vi "qFED.vi"(0 "System no.":i32=1 min=1 max=4 step=1, 2 "Axes to query":string[](array[string]), 3 "All axes?":bool, 4 "Axis identifier?":bool, 5 "error in":errorcluster) -> (14 "Edge ID":i32[](array[numeric]), 15 "Parameter":dbl[](array[numeric]), 19 "error out":errorcluster)   [LabVIEW 2026]
doc: "Get the parameters of the last Find Edge motion performed with FED.\n\nC-843: If All axes? = TRUE, then Axis identifier? can be FALSE"
panel:
  # "Get the parameters of the last Find Edge motion performed with FED."
  # "If all axes: use"
  # "Query"
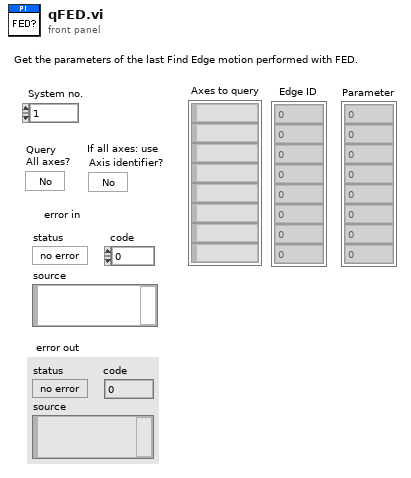
[diagram p1: front panel]
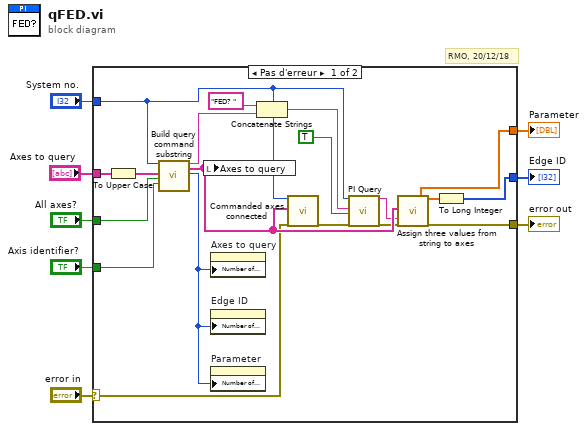
[diagram p0: block diagram]
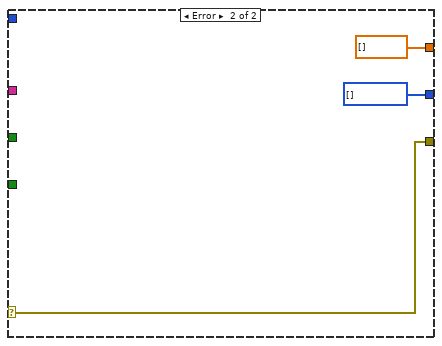
[diagram p2: hidden frame]
diagram:
  # "RMO, 20/12/18"
  n1 = case shown="Pas d'erreur" "error in" {
    selector: "error in" -> [w12 w28]
    tunnel: "Axes to query" -> [w25 _]
    tunnel: "System no." -> [w11 _]
    tunnel: [w27 w28] -> w6
    tunnel: [w15 i32[] [] ("Parameter values")] -> w5
    tunnel: [w14 dbl[] [] ("Source ID")] -> w4
    tunnel: "All axes?" -> [w24 _]
    tunnel: "Axis identifier?" -> [w23 _]
    frame No Error {
      n2 = To Upper Case(1:w25) -> (0:w26:string[])
      n3 = call "Build query command substring.vi"("System no."=w11, "Axes to query in"=w26, "Query\nAll axes?"=w24, "For all axes: use\nAxis identifier?"=w23) -> ("Command substring"=w18:string, "Axes to query out"=w13:string[], "Number of rows"=w22:u32)  [unwired: 2 in, 11 out]
      n4 = local write "Axes to query"(w13) -> ()
      n5 = property on="Axes to query" class="Tabl (strict)"("Number of Rows"=w22) -> ()  [unwired: 2 in, 2 out]
      n6 = property on="Edge ID" class="Tabl (strict)"("Number of Rows"=w22) -> ()  [unwired: 2 in, 2 out]
      n7 = property on="Parameter" class="Tabl (strict)"("Number of Rows"=w22) -> ()  [unwired: 2 in, 2 out]
      n8 = Concatenate Strings("FED? ", w18) -> (w20:string)
      n9 = call "Commanded axes connected.vi"("System no."=w11, "Commanded axes"=w13, "error in"=w12) -> ("error out"=w17:errorcluster)  [unwired: 1 in, 15 out]
      n10 = call "PI Query.vi"("System no."=w11, "String to send"=w20, "Attach termination char.?"=TRUE ("Attach Linefeed?"), "error in"=w17) -> ("String read"=w9:string, "error out"=w10:errorcluster)  [unwired: 3 in, 11 out]
      n11 = call "Assign three values from string to axes.vi"("Queried axes"=w13, "Input String"=w9, "error in"=w10) -> ("Values 2"=w14:dbl[], "Values 1"=w16:dbl[], "error out"=w27:errorcluster)  [unwired: 14 out]
      n12 = To Long Integer(number=w16) -> (32bit integer=w15:i32[])
    }
    frame Error {
    }
  }
  "Parameter" <- w4
  "error out" <- w6
  "Edge ID" <- w5
